vi "SR.vi"(4 "Reset":bool, 5 "Set":bool) -> (1 "Out":bool)   [LabVIEW 2020]
panel:
  out "Mem":bool
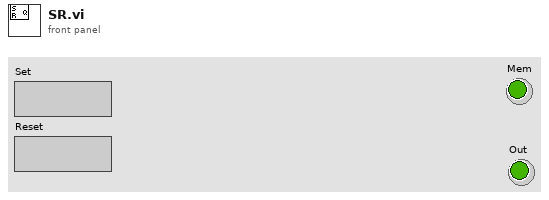
[diagram p1: front panel]
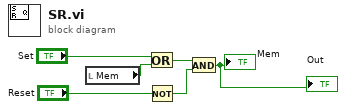
[diagram p0: block diagram]
diagram:
  n1 = local read "Mem"() -> (w2:bool)
  n2 = Or(x="Set", y=w2) -> (x .or. y?=w5:bool)
  n3 = Not(x="Reset") -> (.not. x?=w3:bool)
  n4 = And(x=w5, y=w3) -> (x .and. y?=→"Mem" →"Out":bool)
